vi "Agilent SNA Read Power.vi"(4 "Passthrough (T)":bool=TRUE, 6 "Channel":i8=1 min=1 max=99 step=1, 7 "Agilent SNA & SWP":T1, 8 "error in (no error)":errorcluster, 11 "VISA Resource Names":T2) -> (0 "error out":errorcluster, 2 "Source Power, dBm":dbl, 3 "dup VISA Resource Names":T2)   [LabVIEW 2011]
doc: "This vi sets the power range. Only works on the HP 8753D."
uses:
  TypeDefs/Agilent SNA VISA.ctl
  TypeDefs/Agilent SNA Instrument Info.ctl
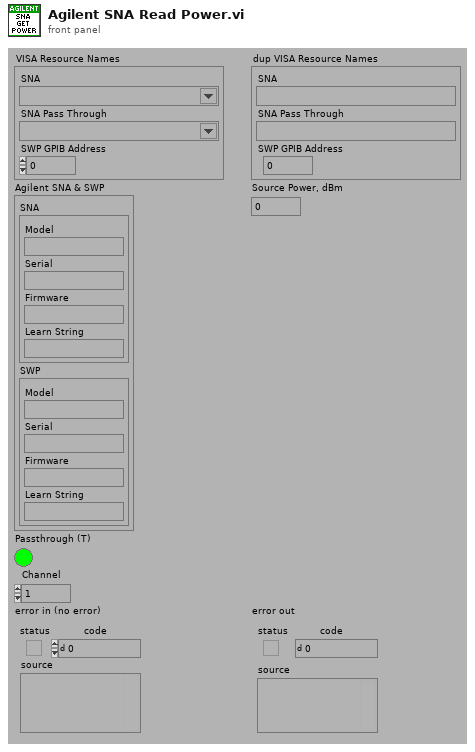
[diagram p1: front panel]
types:
  T1 = typedef "Agilent SNA Instrument Info.ctl" = cluster{"SNA":cluster{"Model":string, "Serial":string, "Firmware":string, "Learn String":string}, "SWP":cluster{"Model":string, "Serial":string, "Firmware":string, "Learn String":string}}
  T2 = typedef "Agilent SNA VISA.ctl" = cluster{"SNA":refnum<visa-resource-name>, "SNA Pass Through":refnum<visa-resource-name>, "SWP GPIB Address":i32}
  T3 = typedef "Agilent SNA Model.ctl" = enum16{"Not Supported", "8757X"}
  T4 = typedef "Agilent SNA SWP Model.ctl" = enum16{"Not Supported", "836XXX", "8375XX", "E82X7D"}
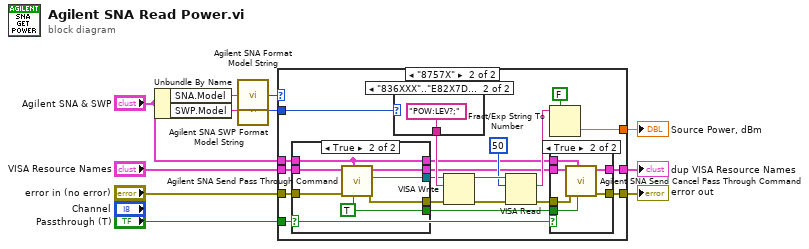
[diagram p0: block diagram]
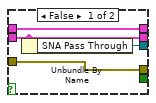
[diagram p4: hidden frame]
diagram:
  n1 = Unbundle By Name("Agilent SNA & SWP") -> ("SNA.Model"=w8:string, "SWP.Model"=w5:string)
  n2 = call "Agilent SNA Format Model String.vi"("Model String"=w8) -> ("Model"=w7:T3)
  n3 = call "Agilent SNA SWP Format Model String.vi"("Model String"=w5) -> ("Model"=w4:T4)
  n4 = case shown="\"8757X\"" w7 {
    tunnel: "error in (no error)" -> [w13 w19]
    tunnel: [_ w33] -> w10
    tunnel: [w13 w24] -> w9
    tunnel: "Agilent SNA & SWP" -> [_ w21]
    tunnel: w4 -> [_ w30]
    tunnel: [w12 w25] -> w3
    tunnel: "VISA Resource Names" -> [w12 w20]
    tunnel: "Passthrough (T)" -> [_ w15]
    frame "Not Supported" {
    }
    frame "8757X" {
      n5 = case shown="True" w15 {
        tunnel: [w43 w52] -> w17
        tunnel: w19 -> [w44 w51]
        tunnel: w20 -> [w42 w50]
        tunnel: [w44 w49] -> w18
        tunnel: w21 -> [w45 w46]
        tunnel: [w42 w48] -> w16
        tunnel: [_ w47] -> w14
        tunnel: [w45 w46] -> w22
        frame False {
          n6 = Unbundle By Name(w42) -> ("SNA Pass Through"=w43:refnum<visa-resource-name>)
        }
        frame True {
          w47 = TRUE ("SCPI? (F)")
          n7 = call "Agilent SNA Send Pass Through Command.vi"("SCPI? (F)"=w47, "Agilent SNA & SWP"=w46, "error in (no error)"=w51, "VISA Resource Names"=w50) -> ("error out"=w49:errorcluster, "SNA Pass Through"=w52:refnum<visa-resource-name>, "dup VISA Resource Names"=w48:T2)  [unwired: 5 out]
        }
      }
      n8 = case shown="\"836XXX\"..\"E82X7D\"" w30 {
        tunnel: [_ "POW:LEV?;"] -> w31
        frame "Not Supported" {
        }
        frame "836XXX".."E82X7D" {
        }
      }
      n9 = VISA Write(VISA resource name=w17, write buffer=w31, error in (no error)=w18) -> (VISA resource name out=w28:refnum<visa-resource-name>, error out=w29:errorcluster)  [unwired: 1 out]
      n10 = VISA Read(VISA resource name=w28, byte count=u32 50, error in (no error)=w29) -> (read buffer=w26:string, error out=w23:errorcluster)  [unwired: 2 out]
      n11 = Fract/Exp String To Number(use system decimal point (T)=FALSE, string=w26) -> (number=w33:dbl)  [unwired: 3 out]
      n12 = case shown="True" w15 {
        tunnel: [w35 w41] -> w24
        tunnel: w16 -> [w34 w40]
        tunnel: w23 -> [w35 w39]
        tunnel: [w34 w38] -> w25
        tunnel: w22 -> [_ w37]
        tunnel: w14 -> [_ w36]
        frame False {
        }
        frame True {
          n13 = call "Agilent SNA Send Cancel Pass Through Command.vi"("SCPI? (F)"=w36, "Agilent SNA & SWP"=w37, "error in (no error)"=w39, "VISA Resource Names"=w40) -> ("error out"=w41:errorcluster, "dup VISA Resource Names"=w38:T2)  [unwired: 6 out]
        }
      }
    }
  }
  "dup VISA Resource Names" <- w3
  "error out" <- w9
  "Source Power, dBm" <- w10
